vi "openCPC3725.vi"(8 "error in (no error)":errorcluster, 11 "CPC IP":string="169.254.70.41") -> (0 "error out":errorcluster, 3 "connection ID":refnum<k5>)   [LabVIEW 2017]
doc: "Use this template to build a VI to use as a subVI."
panel:
  out "data out 4":string
  out "data out 3":string
  out "value":T1
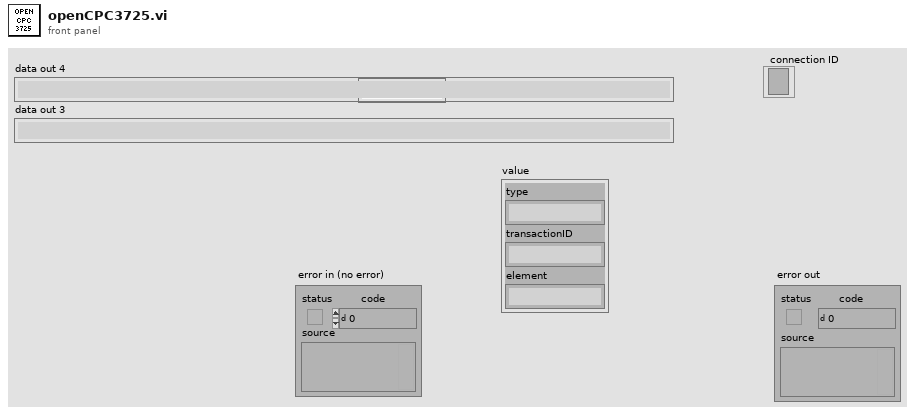
[diagram p1: front panel]
types:
  T1 = cluster{"type":string, "transactionID":string, "element":string}
  T2 = enum16{"Standard", "Buffered", "CRLF", "Immediate"}
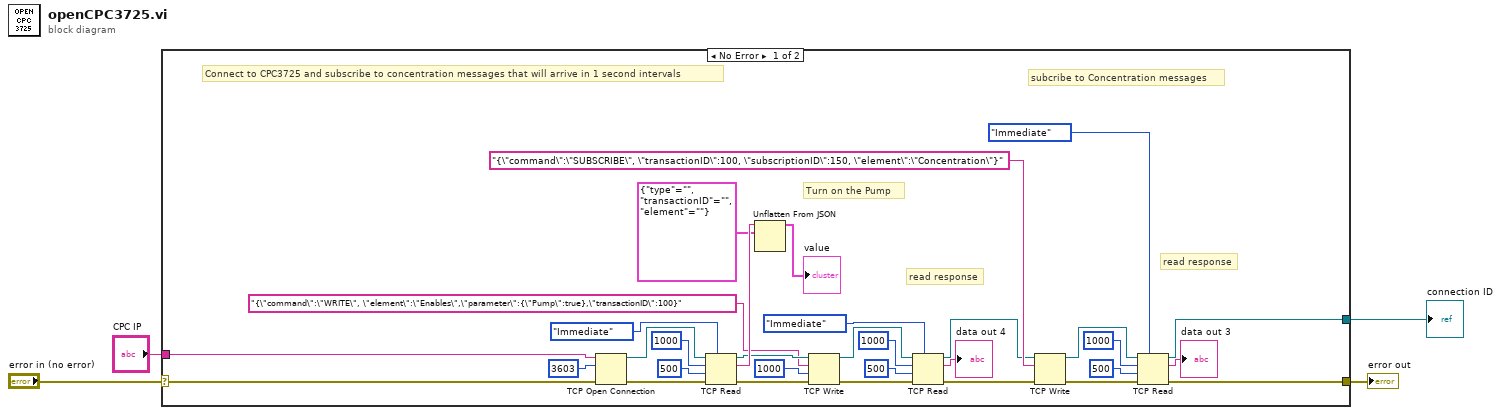
[diagram p0: block diagram]
diagram:
  n1 = case shown="No Error" "error in (no error)" {
    selector: "error in (no error)" -> [w7 w37]
    tunnel: [w6 w37] -> w3
    tunnel: "CPC IP" -> [w8 _]
    tunnel: [w5 _] -> w1
    frame No Error {
      # "Connect to CPC3725 and subscribe to concentration messages that will arrive in 1 second intervals"
      # "read response"
      # "read response"
      # "subcribe to Concentration messages"
      # "Turn on the Pump"
      n2 = TCP Open Connection(address=w8, remote port or service name=u16 3603, error in (no error)=w7) -> (connection ID=w34:refnum<k5>, error out=w35:errorcluster)  [unwired: 2 in]
      n3 = TCP Read(connection ID=w34, bytes to read=1000, error in (no error)=w35, 7:T2."Immediate" ("mode (standard)"), 9:500 ("timeout ms (25000)")) -> (connection ID out=w27:refnum<k5>, data out=w30:string, error out=w26:errorcluster)
      n4 = Unflatten From JSON(JSON string=w30, type and defaults=T1 {"type"="", "transactionID"="", "element"=""}) -> (value=→"value":T1)  [unwired: 5 in, 1 out]
      n5 = TCP Write(connection ID=w27, data in="{\"command\":\"WRITE\", \"element\":\"Enables\",\"parameter\":{\"Pump\":true},\"transactionID\":100}", error in (no error)=w26, 9:1000 ("timeout ms (25000)")) -> (connection ID out=w13:refnum<k5>, error out=w15:errorcluster)  [unwired: 1 out]
      n6 = TCP Read(connection ID=w13, bytes to read=1000, error in (no error)=w15, 7:T2."Immediate" ("mode (standard)"), 9:500 ("timeout ms (25000)")) -> (connection ID out=w12:refnum<k5>, data out=→"data out 4":string, error out=w14:errorcluster)
      n7 = TCP Write(connection ID=w12, data in="{\"command\":\"SUBSCRIBE\", \"transactionID\":100, \"subscriptionID\":150, \"element\":\"Concentration\"}", error in (no error)=w14) -> (connection ID out=w22:refnum<k5>, error out=w9:errorcluster)  [unwired: 1 in, 1 out]
      n8 = TCP Read(connection ID=w22, bytes to read=1000, error in (no error)=w9, 7:T2."Immediate" ("mode (standard)"), 9:500 ("timeout ms (25000)")) -> (connection ID out=w5:refnum<k5>, data out=→"data out 3":string, error out=w6:errorcluster)
    }
    frame Error {
    }
  }
  "error out" <- w3
  "connection ID" <- w1
